vi "Simple Read.vi"(4 "Abs_I8 Integer in":refnum<class "Abs_I8 Integer.lvclass">) -> (1 "Value":i8)   [LabVIEW 2021, in "Abs_I8 Integer.lvclass"]
uses:
  Abs_I8 Integer.lvclass
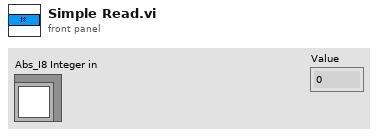
[diagram p1: front panel]
types:
  T1 = typedef "Abs_I8 Integer.lvclass/Type.ctl" = i8
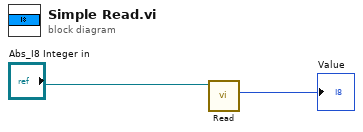
[diagram p0: block diagram]
diagram:
  n1 = call-dynamic "Read.vi"("Double Float.lvclass_340760 in"="Abs_I8 Integer in") -> ("Value"=→"Value":T1)  [unwired: 8 in, 2 out]
